vi "Untitled 1.vi"   [LabVIEW 2018]
uses:
  <vilib>/Platform/TimedLoop/XDataNode/XDataNode.xnode
  <vilib>/Platform/TimedLoop/XDataNode/timing_clust.ctl
  <vilib>/Platform/TimedLoop/XDataNode/XDNodeRunTimeDep.lvlib
  <vilib>/Platform/TimedLoop/XDataNode/wakeup.ctl
  <vilib>/Platform/TimedLoop/XDataNode/nitl_modes.ctl
types:
  T1 = typedef "XDNodeRunTimeDep.lvlib/timing_clust.ctl" = cluster{"Expected End [f-1]":u64, "Actual End [f-1]":u64, "Finished Late? [f-1]":bool, "Expected End [i-1]":u64, "Actual End [i-1]":u64, "Finished Late? [i-1]":bool, "Expected Start [i]":u64, "Actual Start [i]":u64, "Expected Start [f]":u64, "Actual Start [f]":u64, "Source Name":string, "Structure Name":string, "Period":i64, "Deadline":i64, "Offset":i64, "Start":i64, "Priority":i32, "Timeout":i32, "Mode":T2, "Wakeup Reason":T3, "Error":errorcluster, "Source Type":string, "Secondary Source Type":string, "Global End Time":u64, "Global Start Time":u64, "Frame Duration":u64, "Iteration Duration":u64, "Assigned CPU":i32, "I/O Scan Engine Mode":u32}
  T2 = typedef "XDNodeRunTimeDep.lvlib/nitl_modes.ctl" = enum32{"No Change", "Process missed periods, maintain original phase", "Discard missed periods, maintain original phase", "Process missed periods, ignore original phase", "Discard missed periods, ignore original phase"}
  T3 = typedef "XDNodeRunTimeDep.lvlib/wakeup.ctl" = enum32{"Normal", "Aborted", "Asynchronous wakeup", "Timing source error", "Timed loop error", "Timeout"}
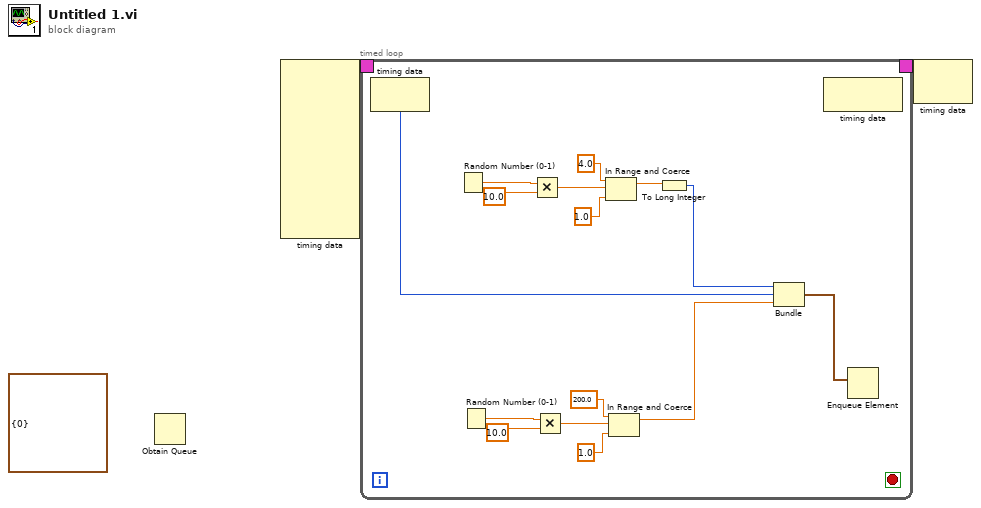
[diagram p0: block diagram]
diagram:
  (unwired) cluster{i32} {0}
  n1 = Obtain Queue() -> ()  [unwired: 5 in, 3 out]
  n2 = node-c288() -> (w2:T1)  [unwired: 10 in]
  n3 = timed-loop {
    timing: w2 -> [_]
    timing-out: [_] -> w1
    stop <- _ stop-if-true
    n4 = node-c288() -> (w4:i64)  [unwired: 1 in]
    n5 = Random Number (0-1)() -> (number: 0 to 1=w17:dbl)
    n6 = Random Number (0-1)() -> (number: 0 to 1=w12:dbl)
    n7 = Multiply(x=w17, y=10.0) -> (x*y=w15:dbl)
    n8 = Multiply(x=w12, y=10.0) -> (x*y=w10:dbl)
    n9 = In Range and Coerce(upper limit=4.0, x=w15, lower limit=1.0) -> (coerced(x)=w7:dbl)  [unwired: 1 out]
    n10 = In Range and Coerce(upper limit=200.0, x=w10, lower limit=1.0) -> (coerced(x)=w5:dbl)  [unwired: 1 out]
    n11 = To Long Integer(number=w7) -> (32bit integer=w6:i32)
    n12 = Bundle(w6, "Period"=w4, "upper limit"=w5) -> (w3:cluster{i32, "Period":i64, "upper limit":dbl})  [unwired: 1 in]
    n13 = node-c288() -> ()  [unwired: 1 in, 1 out]
    n14 = Enqueue Element(element=w3) -> ()  [unwired: 3 in, 3 out]
  }
  n15 = node-c288(w1) -> ()  [unwired: 1 out]
